vi "create new cluster centers.vi"(0 "Pattern (0) Distance data (1-4) cluster (5) output":string[][](array[string]), 2 "Old cluster centers":string[](array[string])) -> (7 "New cluster centers":string[](array[string]))   [LabVIEW 2013]
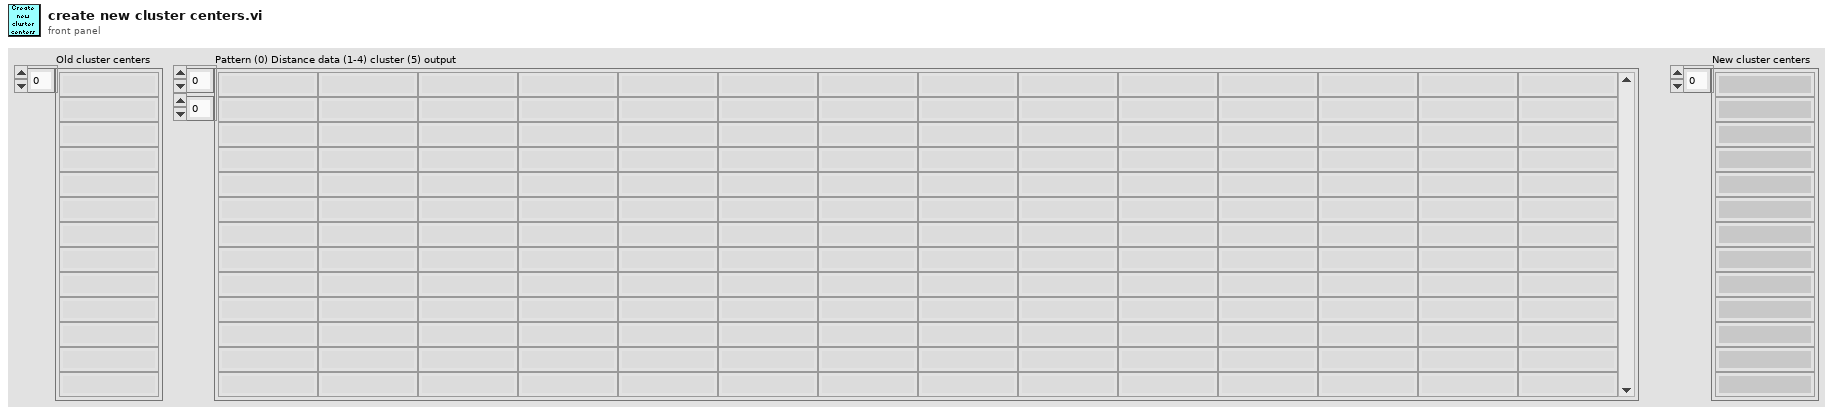
[diagram p1: front panel]
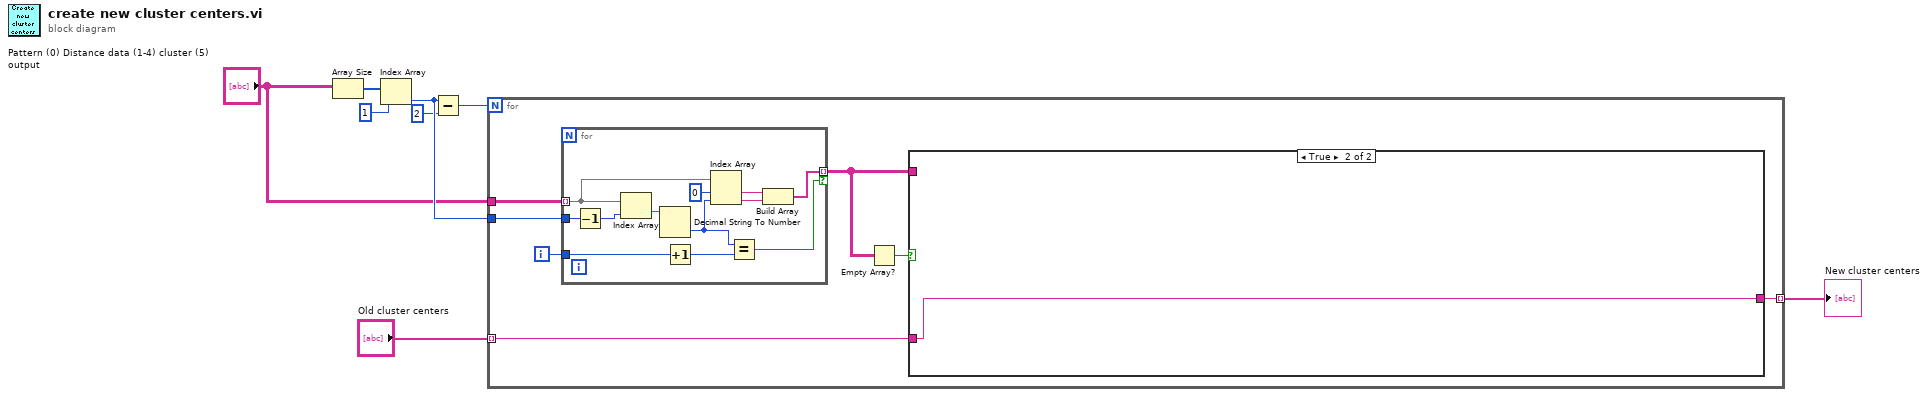
[diagram p0: block diagram]
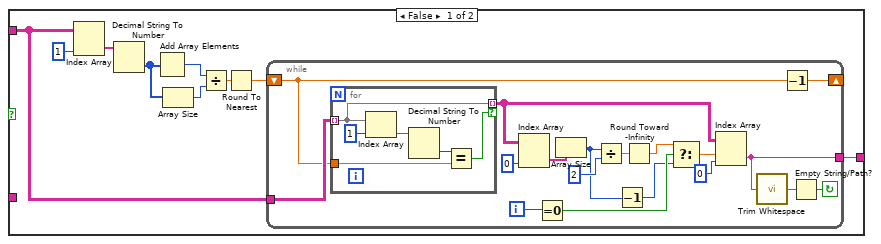
[diagram p2: hidden frame]
diagram:
  n1 = Array Size(array="Pattern (0) Distance data (1-4) cluster (5) output") -> (size(s)=w4:i32[])
  n2 = Index Array(array=w4, index=1) -> (element=w8:i32)
  n3 = Subtract(x=w8, y=2) -> (x-y=w7:i32)
  n4 = for {
    N: w7 -> [_]
    tunnel: "Pattern (0) Distance data (1-4) cluster (5) output" -> [w15]
    tunnel: w8 -> [w14]
    tunnel: [w12] -> w3 mode=indexing
    tunnel: "Old cluster centers" -> [w9] mode=indexing
    i -> [w13]
    n5 = for {
      tunnel: w15 -> [w56] mode=indexing
      tunnel: w14 -> [w60]
      tunnel: w13 -> [w54]
      tunnel: [w51] -> w11 mode=indexing if=w50
      n6 = Decrement(x=w60) -> (x-1=w61:i32)
      n7 = Index Array(array=w56, index=w61) -> (element=w55:string)
      n8 = Decimal String To Number(string=w55) -> (number=w52:i32)  [unwired: 2 in, 1 out]
      n9 = Increment(x=w54) -> (x+1=w53:i32)
      n10 = Index Array(array=w56, index #1=0 ("index"), index #2=w52) -> (element #1=w58:string, element #2=w59:string)
      n11 = Equal?(x=w52, y=w53) -> (x = y?=w50:bool)
      n12 = Build Array(w58, w59) -> (w51:string[])
    }
    n13 = Empty Array?(array=w11) -> (empty?=w10:bool)
    n14 = case shown="True" w10 {
      tunnel: [w17 w49] -> w12
      tunnel: w11 -> [w16 _]
      tunnel: w9 -> [_ w49]
      frame False {
        n15 = Index Array(array=w16, index (col)=1 ("disabled index (col)")) -> (element=w23:string[])  [unwired: 1 in]
        n16 = Decimal String To Number(string=w23) -> (number=w22:i32[])  [unwired: 2 in, 1 out]
        n17 = Add Array Elements(numeric array=w22) -> (sum=w21:i32)
        n18 = Array Size(array=w22) -> (size(s)=w20:i32)
        n19 = Divide(x=w21, y=w20) -> (x/y=w19:dbl)
        n20 = Round To Nearest(number=w19) -> (nearest integer value=w18:dbl)
        n21 = while {
          tunnel: w16 -> [w36]
          tunnel: [w35] -> w17
          shift-right: [w32] -> _
          shift-left: w18 -> [w31]
          i -> [w28]
          stop <- w33 continue-if-true
          n22 = for {
            tunnel: w36 -> [w45] mode=indexing
            tunnel: [w45] -> w41 mode=indexing if=w44
            tunnel: w31 -> [w43]
            n23 = Index Array(array=w45, index=1) -> (element=w47:string)
            n24 = Decimal String To Number(string=w47) -> (number=w46:i32)  [unwired: 2 in, 1 out]
            n25 = Equal?(x=w46, y=w43) -> (x = y?=w44:bool)
          }
          n26 = Index Array(array=w41, index (col)=0 ("disabled index (col)")) -> (element=w37:string[])  [unwired: 1 in]
          n27 = Equal To 0?(x=w28) -> (x = 0?=w26:bool)
          n28 = Array Size(array=w37) -> (size(s)=w30:i32)
          n29 = Divide(x=w30, y=2) -> (x/y=w40:dbl)
          n30 = Decrement(x=w30) -> (x-1=w25:i32)
          n31 = Round Toward -Infinity(1:w40) -> (0:w27:dbl)
          n32 = Select(t=w27, s=w26, f=w25) -> (s? t:f=w29:dbl)
          n33 = Index Array(array=w41, index (row)=w29, index (col)=0 ("disabled index (col)")) -> (element=w35:string)
          n34 = call <vilib>:"Trim Whitespace.vi"("string"=w35) -> ("trimmed string"=w34:string)  [unwired: 1 in]
          n35 = Decrement(x=w31) -> (x-1=w32:dbl)
          n36 = Empty String/Path?(string/path=w34) -> (empty?=w33:bool)
        }
      }
      frame True {
      }
    }
  }
  "New cluster centers" <- w3
